vi "Square wave.vi"() -> ()   [LabVIEW 2020]
panel:
  in  "Slope":bool
  in  "Slope Count":i32=25
  in  "PWM":i32=48000
  in  "Cycle":i32=1
  in  "Freq":i32=160
  out "웨이브폼 그래프":dbl[](graph)
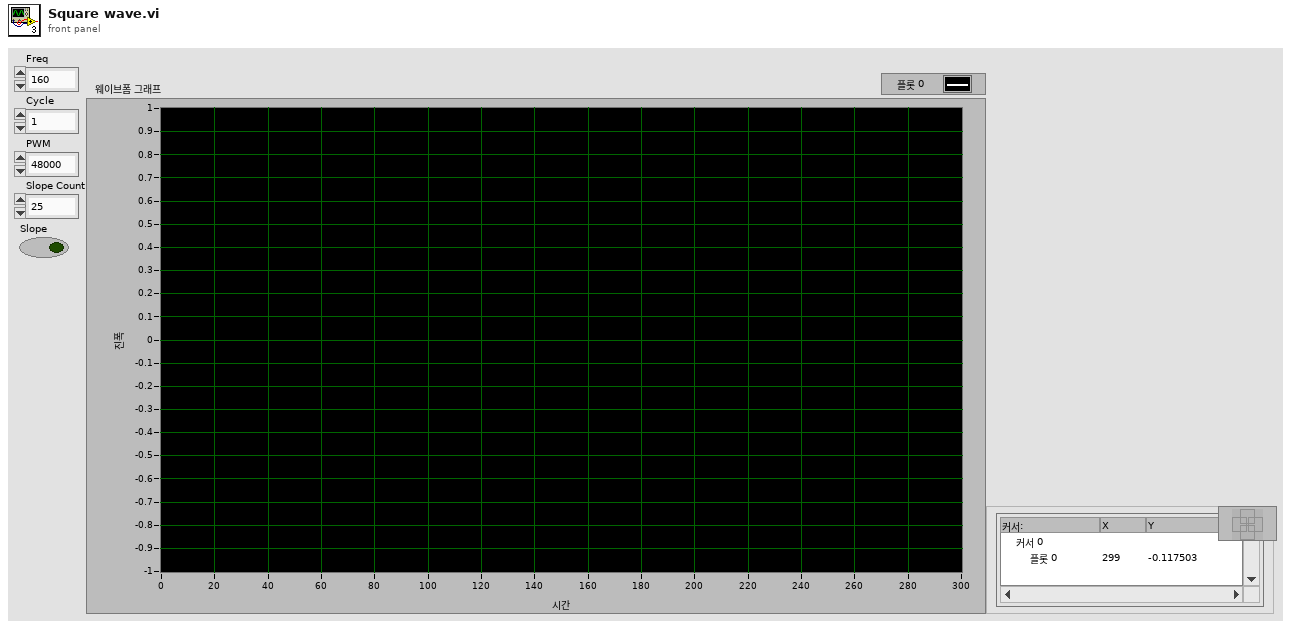
[diagram p1: front panel]
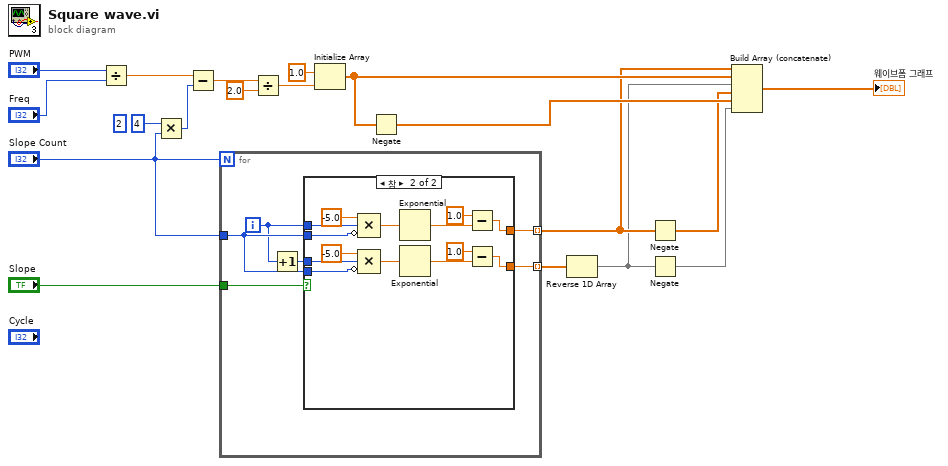
[diagram p0: block diagram]
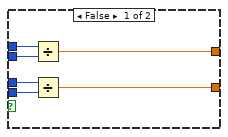
[diagram p2: hidden frame]
diagram:
  (unwired) 2 ("y")
  n1 = Divide(x="PWM", y="Freq") -> (x/y=w16:dbl)
  n2 = Multiply(x=4, y="Slope Count") -> (x*y=w14:i32)
  n3 = Subtract(x=w16, y=w14) -> (x-y=w13:dbl)
  n4 = for {
    N: "Slope Count" -> [_]
    tunnel: "Slope" -> [w25]
    tunnel: "Slope Count" -> [w23]
    tunnel: [w24] -> w5 mode=indexing
    tunnel: [w20] -> w2 mode=indexing
    i -> [w22]
    n5 = Increment(x=w22) -> (x+1=w21:i32)
    n6 = case shown="참" w25 {
      tunnel: w22 -> [w31 w43]
      tunnel: w23 -> [w30 w42]
      tunnel: [w29 w39] -> w24
      tunnel: w23 -> [w27 w34]
      tunnel: w21 -> [w28 w33]
      tunnel: [w26 w32] -> w20
      frame False {
        n7 = Divide(x=w31, y=w30) -> (x/y=w29:dbl)
        n8 = Divide(x=w28, y=w27) -> (x/y=w26:dbl)
      }
      frame True {
        n9 = Compound Arithmetic op=MULTIPLY(-5.0 ("x"), w43, invert w42) -> (w41:dbl)
        n10 = Compound Arithmetic op=MULTIPLY(-5.0 ("x"), w33, invert w34) -> (w37:dbl)
        n11 = Exponential(1:w41) -> (0:w40:dbl)
        n12 = Exponential(1:w37) -> (0:w38:dbl)
        n13 = Subtract(x=1.0, y=w40) -> (x-y=w39:dbl)
        n14 = Subtract(x=1.0, y=w38) -> (x-y=w32:dbl)
      }
    }
  }
  n15 = Divide(x=w13, y=2.0) -> (x/y=w11:dbl)
  n16 = Initialize Array(1.0 ("원소"), w11) -> (w9:dbl[])
  n17 = Negate(x=w9) -> (-x=w8:dbl[])
  n18 = Reverse 1D Array(array=w2) -> (reversed array=w1:dbl[])
  n19 = Negate(x=w5) -> (-x=w4:dbl[])
  n20 = Negate(x=w1) -> (-x=w3:dbl[])
  n21 = Build Array (concatenate)(w5, w9, w1, w4, w8, w3) -> (→"웨이브폼 그래프":dbl[])
